vi "Close ColorProcessor.vi"(8 "error in (no error)":errorcluster, 11 "ColorProcessor reference":refnum<k24>) -> (0 "error out":errorcluster)   [LabVIEW 2015]
uses:
  C:/code/ScientificCameraInterfaces/Installer/Scientific Camera Interfaces/LabVIEW/64_bit/Library_X64/Thorlabs.TSI.ColorInterfaces.dll
  code/ScientificCameraInterfaces/Installer/Scientific Camera Interfaces/LabVIEW/64_bit/Library_X64/Thorlabs.TSI.ColorInterfaces.dll
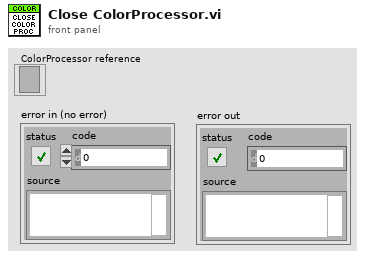
[diagram p1: front panel]
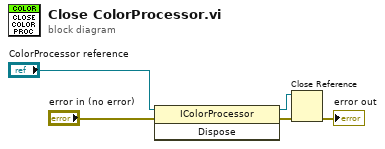
[diagram p0: block diagram]
diagram:
  n1 = invoke class="IColorProcessor" method="Dispose"(reference="ColorProcessor reference", error in="error in (no error)") -> (reference out=w2:refnum<k24>, error out=w3:errorcluster)  [unwired: 1 in, 1 out]
  n2 = Close Reference(reference=w2, error in (no error)=w3) -> (error out=→"error out":errorcluster)
